vi "Unflatten From JSON String.vi"(6 "Nulls as Defaults (F)":bool, 7 "Type and Defaults":variant, 8 "error in (no error)":errorcluster, 11 "JSON String":string) -> (0 "error out":errorcluster, 3 "Variant":variant)   [LabVIEW 2019, in "JKI JSON Serialization.lvlib"]
doc: "Converts <b>JSON String</b> to <b>Variant</b>. If <b>Type and Defaults</b> is provided, converts JSON string to the specified type if the type is compatible with the value of the JSON String. For any cluster element in Type and Defaults, the value of the element in Type and Default is used if element with the same name is not present in the JSON String. If <b>Nulls as Defaults </b> is true, returns the default value as provided in Type and Defaults when null value is encountered in input tree.\n\nJKI JSON 1.1.10.37\nTomi Maila - JKI\nCopyright (c) 2017, JKI"
uses:
  JKI JSON Serialization.lvlib
  Deserializer/JSON Deserializer/JSON Deserializer.lvclass
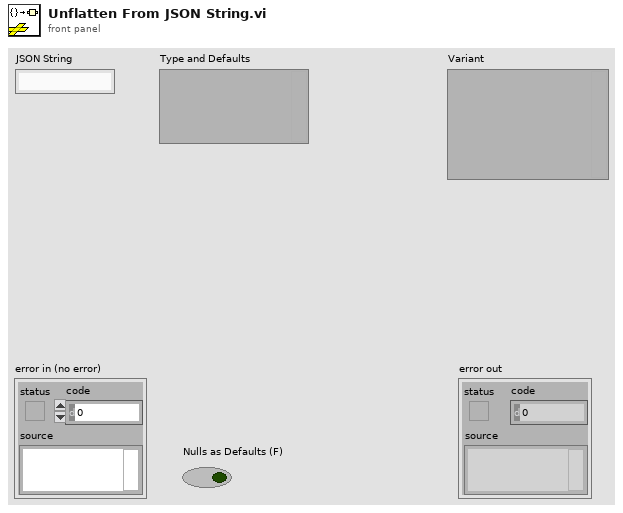
[diagram p1: front panel]
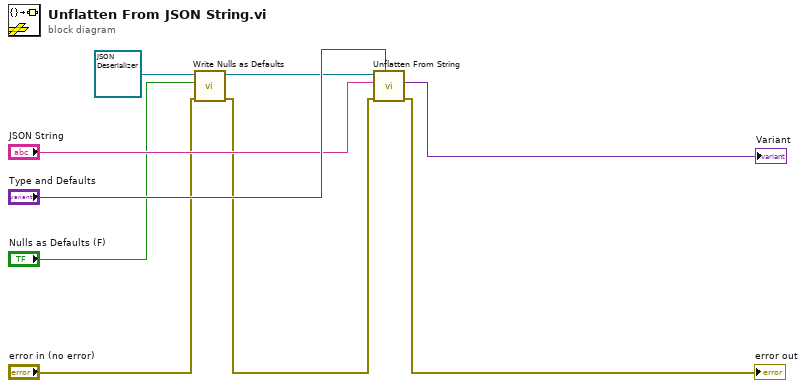
[diagram p0: block diagram]
diagram:
  n1 = call-dynamic "Write Nulls as Defaults.vi"("error in (no error)"="error in (no error)", "Nulls as Defaults"="Nulls as Defaults (F)", "JSON Deserializer in"=refnum<class "JSON Deserializer.lvclass"> refnum ("Deserializer in")) -> ("error out"=w2:errorcluster, "JSON Deserializer out"=w4:refnum<class "JSON Deserializer.lvclass">)  [unwired: 7 in]
  n2 = call-dynamic "Unflatten From String.vi"("Type and Defaults"="Type and Defaults", "error in (no error)"=w2, "String"="JSON String", "Deserializer in"=w4) -> ("error out"=→"error out":errorcluster, "Variant"=→"Variant":variant)  [unwired: 5 in, 1 out]
